vi "Transmitter HMI Main.vi"() -> ()   [LabVIEW 2025]
uses:
  Globals/Cancelled Global.vi
  Globals/Solenoid VISA Global.vi
  <vilib>/Instr/_visa.llb/VISA Configure Serial Port (Instr).vi
  Globals/Touch VISA Global.vi
  Globals/Light VISA Global.vi
  Globals/Motor VISA Global.vi
  Globals/Speaker VISA Global.vi
  Globals/Wire VISA Global.vi
  Globals/Percent Complete Global.vi
panel:
  in  "Enable Wire":bool
  in  "Enable Speaker":bool
  in  "Enable Motor":bool
  in  "Enable Light":bool
  in  "Enable Touch":bool
  in  "Enable Solenoid":bool
  in  "FREQUENCY CHANGER":bool
  in  "Speaker":bool
  in  "Wire":bool
  out "Start Transmission":bool
  out "Exit":bool
  out "Transmitting":bool
  out "Chosen Text":string
  out "Chosen Image Path":path caption="selected path"
  out "Chosen Transmission Method":u16(ring) items=["Speaker", "Wire", "Motor", "Touch", "Light", "Solenoid"]
  out "Chosen Data Type":u16(ring) items=["Text File", "Image File", "Image", "Text"]
  in  "Cancel Button":bool
  out "Transmission Progress:":dbl(slide) scale=0.0..100.0
  in  "Go":bool
  in  "Motor":bool
  in  "Touch":bool
  in  "Light":bool
  in  "Solenoid":bool
  in  "Image":bool
  in  "Text":bool
  # "TRANSMITTER"
  # "1: Select Data Type:"
  # "2: Select Method of Transmission:"
  # "3: BEGIN"
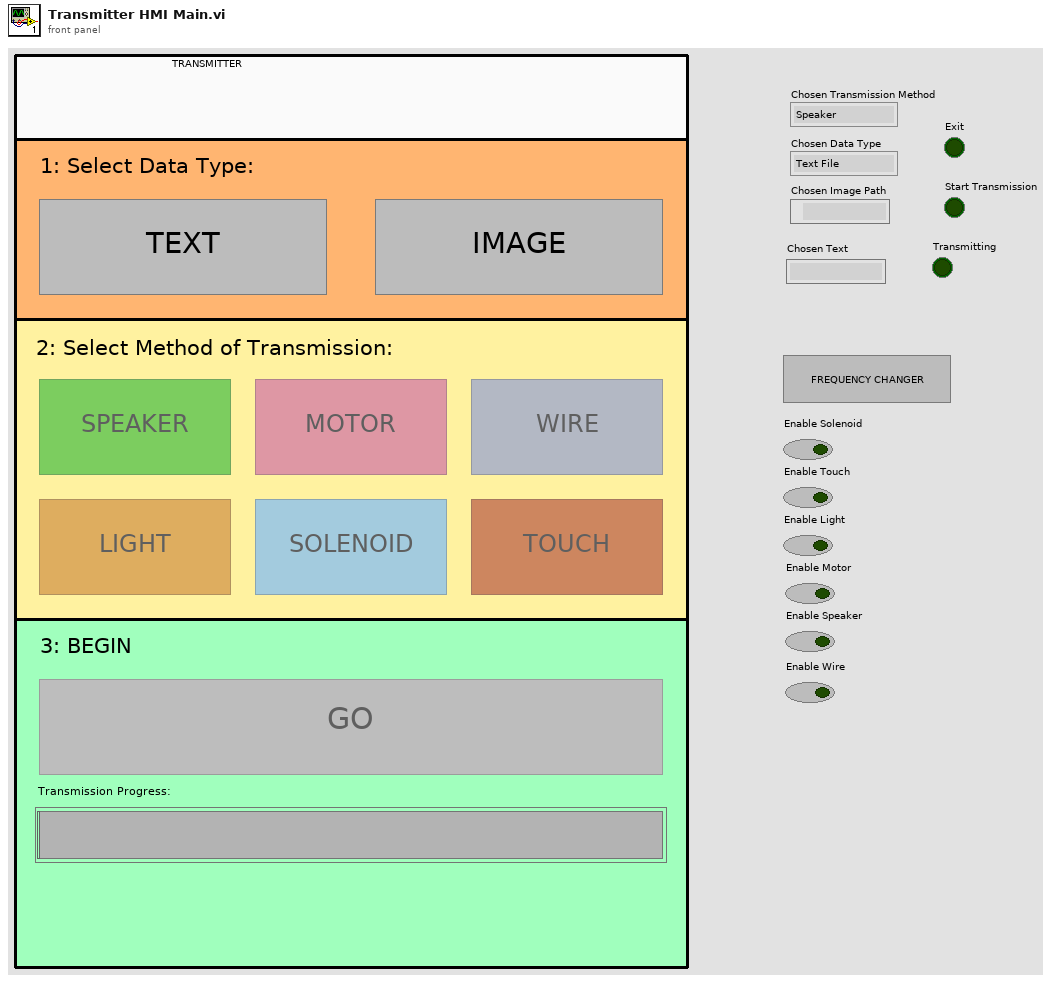
[diagram p1: front panel]
types:
  T1 = enum8{"Enabled", "Disabled", "Disabled and Grayed Out"}
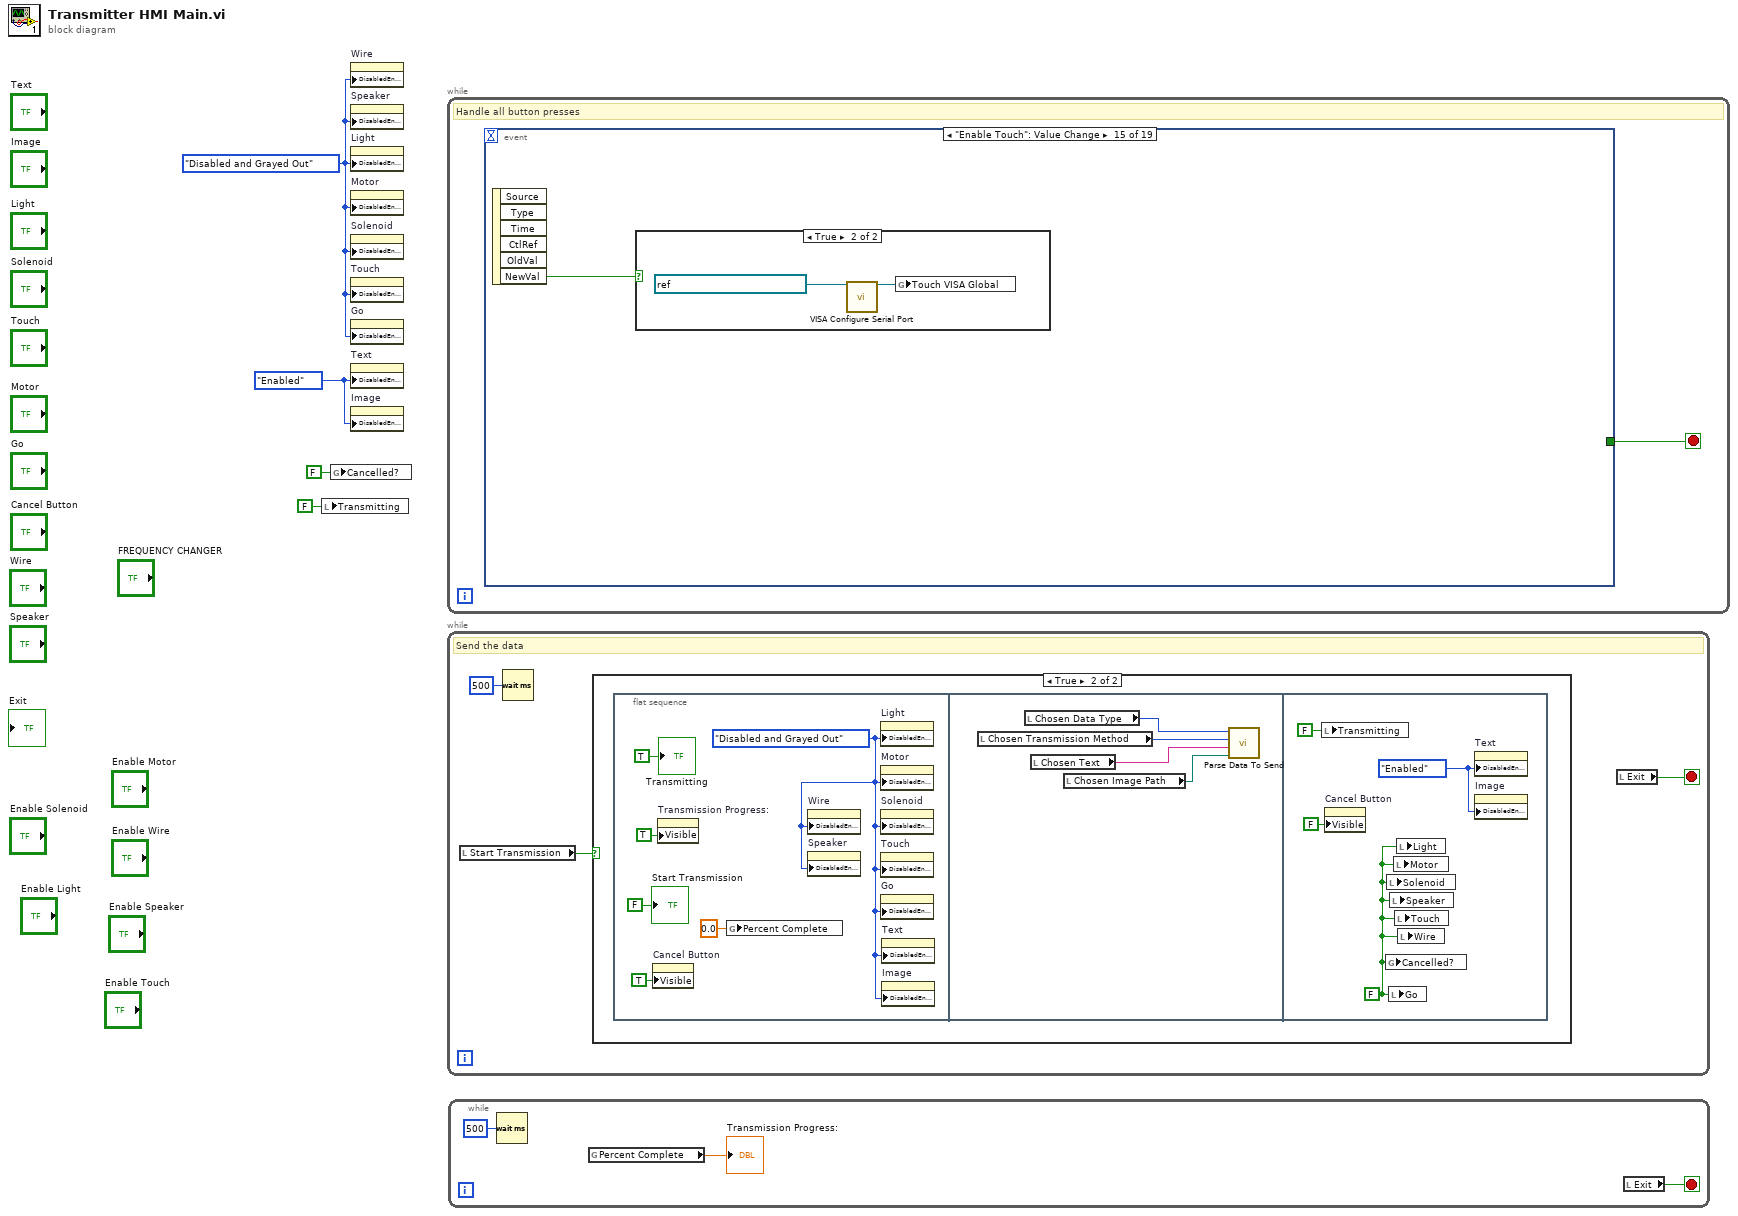
[diagram p0: block diagram]
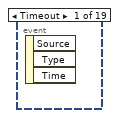
[diagram p3: hidden frame]
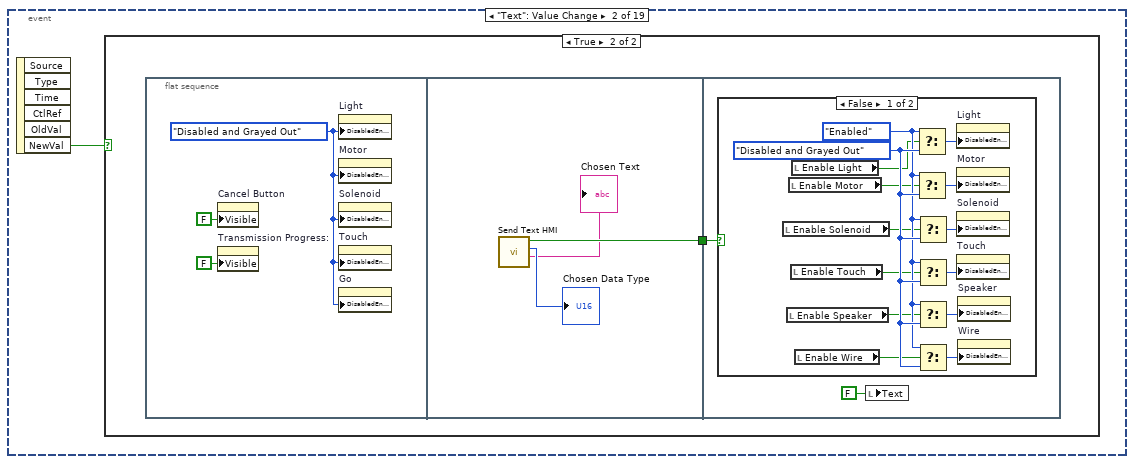
[diagram p4: hidden frame]
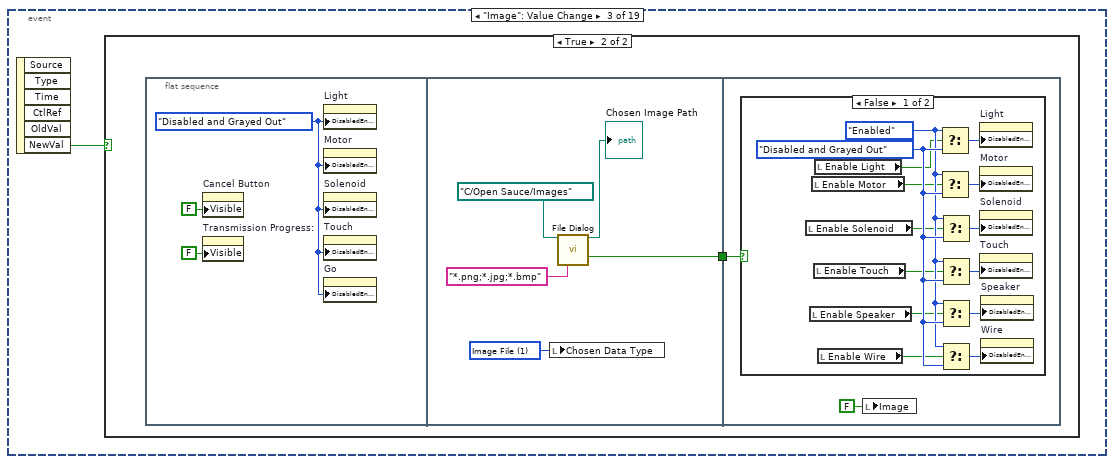
[diagram p7: hidden frame]
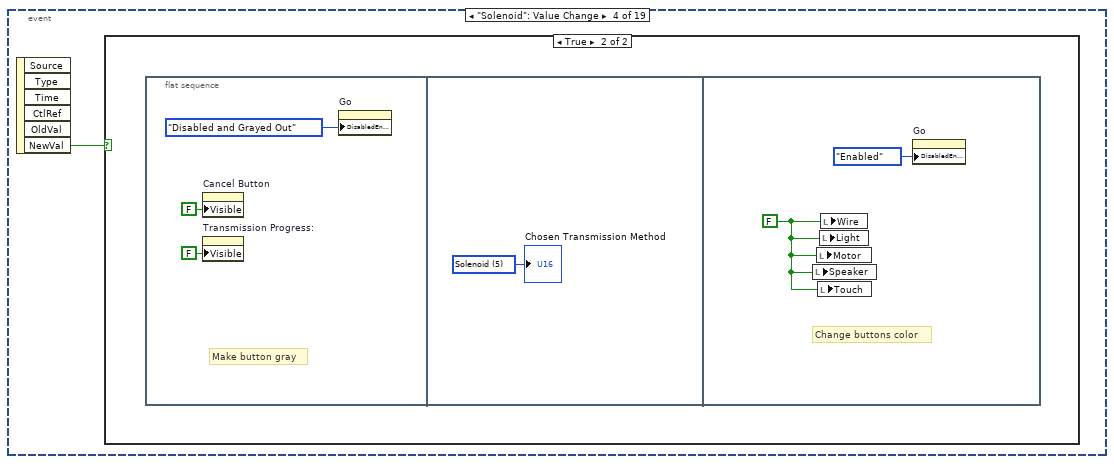
[diagram p10: hidden frame]
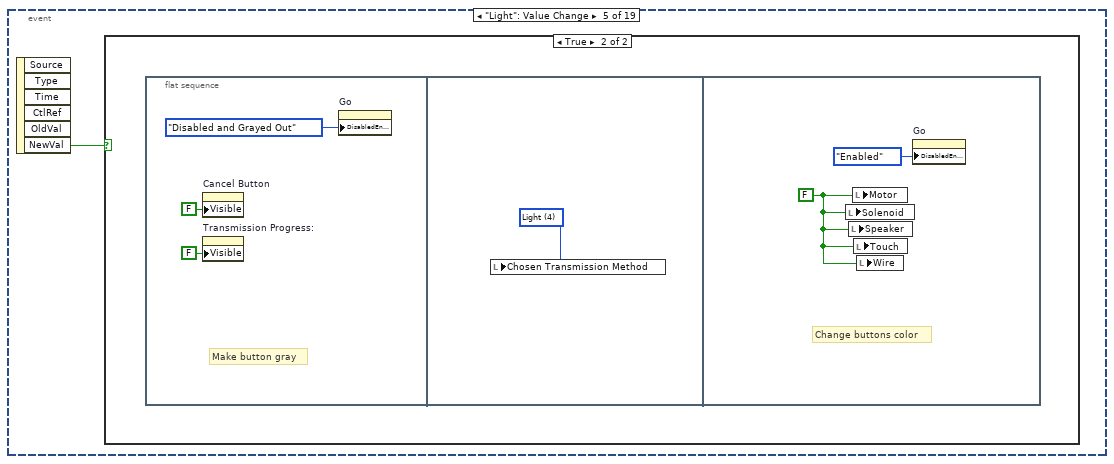
[diagram p12: hidden frame]
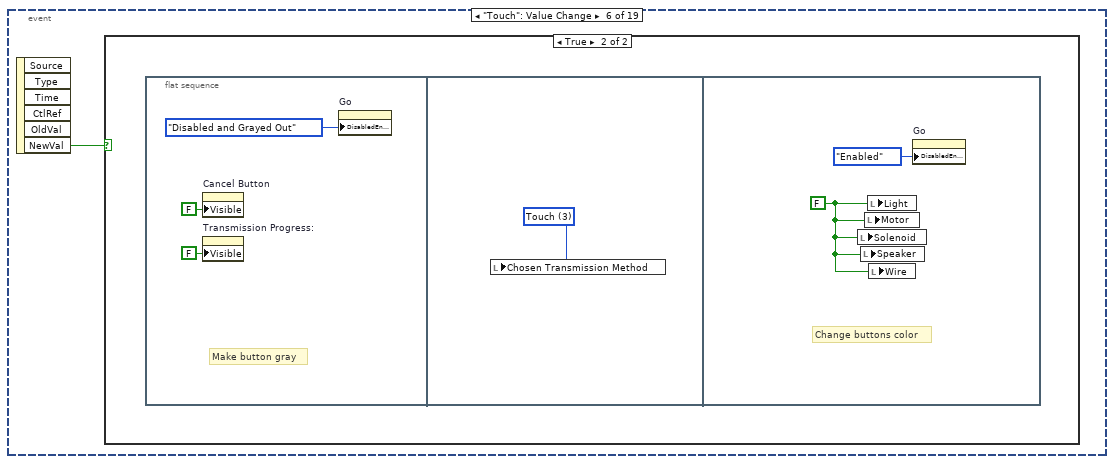
[diagram p14: hidden frame]
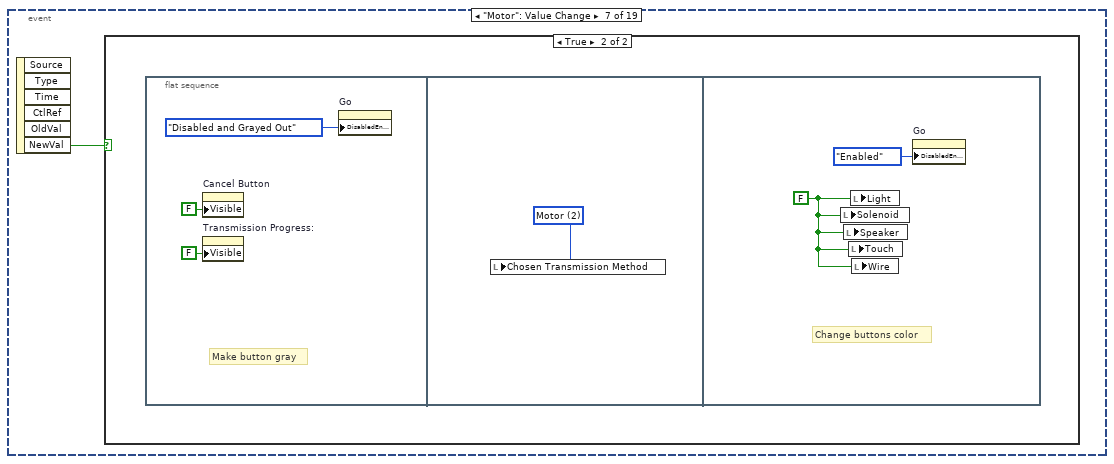
[diagram p16: hidden frame]
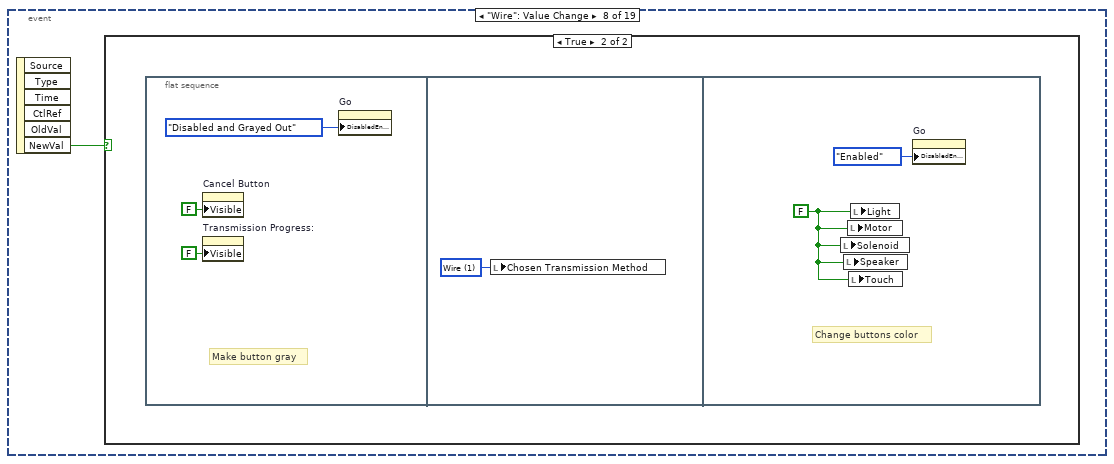
[diagram p18: hidden frame]
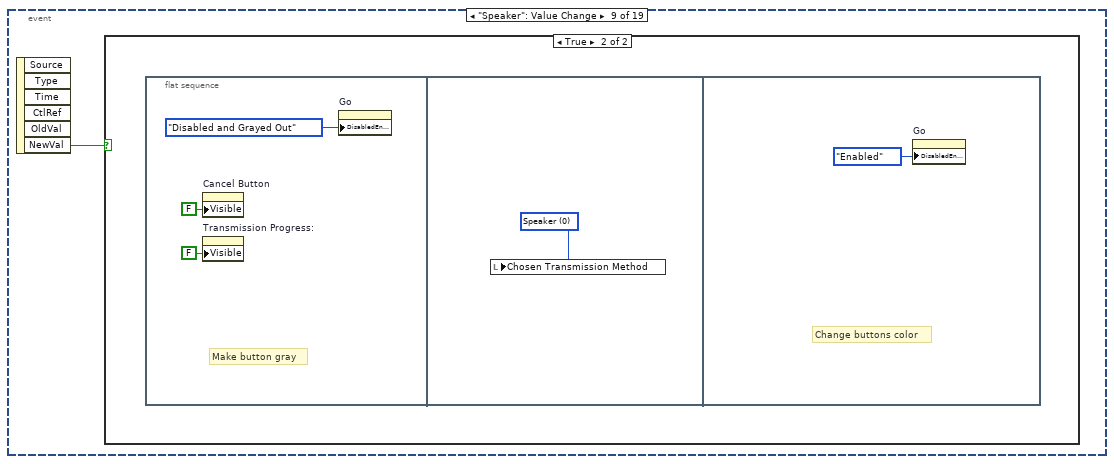
[diagram p20: hidden frame]
diagram:
  w2 = T1."Enabled" ("Disabled")
  w1 = T1."Disabled and Grayed Out" ("Disabled")
  n1 = local write "Transmitting"(FALSE ("Transmitting")) -> ()
  n2 = global write "Cancelled Global.vi" "Cancelled?"(FALSE ("Cancelled?")) -> ()
  n3 = property on="Wire" class="Bool (strict)"("DisabledEnum"=w1) -> ()  [unwired: 2 in, 2 out]
  n4 = property on="Speaker" class="Bool (strict)"("DisabledEnum"=w1) -> ()  [unwired: 2 in, 2 out]
  n5 = property on="Light" class="Bool (strict)"("DisabledEnum"=w1) -> ()  [unwired: 2 in, 2 out]
  n6 = property on="Motor" class="Bool (strict)"("DisabledEnum"=w1) -> ()  [unwired: 2 in, 2 out]
  n7 = property on="Solenoid" class="Bool (strict)"("DisabledEnum"=w1) -> ()  [unwired: 2 in, 2 out]
  n8 = property on="Touch" class="Bool (strict)"("DisabledEnum"=w1) -> ()  [unwired: 2 in, 2 out]
  n9 = property on="Go" class="Bool (strict)"("DisabledEnum"=w1) -> ()  [unwired: 2 in, 2 out]
  n10 = property on="Text" class="Bool (strict)"("DisabledEnum"=w2) -> ()  [unwired: 2 in, 2 out]
  n11 = property on="Image" class="Bool (strict)"("DisabledEnum"=w2) -> ()  [unwired: 2 in, 2 out]
  n12 = while {
    stop <- w5 stop-if-true
    # "Handle all button presses"
    n13 = event shown="[14] \"Enable Touch\": Value Change" {
      selector: _ -> [_ _ _ _ _ _ _ _ _ _ _ _ _ _ _ _ _ _ _]
      dyn-events: _ -> [_ _ _ _ _ _ _ _ _ _ _ _ _ _ _ _ _ _ _]
      timeout: _ -> [_ _ _ _ _ _ _ _ _ _ _ _ _ _ _ _ _ _ _]
      tunnel: [_ _ _ _ _ _ _ _ _ TRUE _ _ _ _ _ _ _ _ _] -> w5
      event Timeout {
        n14 = event-data() -> ()  [unwired: 1 in, 3 out]
      }
      event "Text": Value Change {
        n15 = event-data() -> ("NewVal"=w6:bool)  [unwired: 1 in, 5 out]
        n16 = case shown="True" w6 {
          frame False {
          }
          frame True {
            n17 = flat-sequence {
              tunnel: [w13] -> w7
              tunnel: w7 -> [w15]
              frame #0 {
                w9 = T1."Disabled and Grayed Out" ("Disabled")
                n18 = property on="Cancel Button" class="Bool (strict)"("Visible"=FALSE) -> ()  [unwired: 2 in, 2 out]
                n19 = property on="Transmission Progress:" class="Slide (strict)"("Visible"=FALSE) -> ()  [unwired: 2 in, 2 out]
                n20 = property on="Light" class="Bool (strict)"("DisabledEnum"=w9) -> ()  [unwired: 2 in, 2 out]
                n21 = property on="Motor" class="Bool (strict)"("DisabledEnum"=w9) -> ()  [unwired: 2 in, 2 out]
                n22 = property on="Solenoid" class="Bool (strict)"("DisabledEnum"=w9) -> ()  [unwired: 2 in, 2 out]
                n23 = property on="Touch" class="Bool (strict)"("DisabledEnum"=w9) -> ()  [unwired: 2 in, 2 out]
                n24 = property on="Go" class="Bool (strict)"("DisabledEnum"=w9) -> ()  [unwired: 2 in, 2 out]
              }
              frame #1 {
                n25 = call "Send Text HMI.vi"() -> ("Chosen Text"=→"Chosen Text":string, "Chosen Data Type"=→"Chosen Data Type":u16, "Cancelled"=w13:bool)  [unwired: 9 in]
              }
              frame #2 {
                n26 = case shown="False" w15 {
                  frame False {
                    w23 = T1."Disabled and Grayed Out" ("Disabled")
                    w22 = T1."Enabled" ("Disabled")
                    n27 = local read "Enable Solenoid"() -> (w18:bool)
                    n28 = local read "Enable Speaker"() -> (w20:bool)
                    n29 = local read "Enable Motor"() -> (w17:bool)
                    n30 = local read "Enable Touch"() -> (w19:bool)
                    n31 = local read "Enable Light"() -> (w16:bool)
                    n32 = local read "Enable Wire"() -> (w21:bool)
                    n33 = Select(t=w22, s=w16, f=w23) -> (s? t:f=w29:T1)
                    n34 = Select(t=w22, s=w17, f=w23) -> (s? t:f=w28:T1)
                    n35 = Select(t=w22, s=w18, f=w23) -> (s? t:f=w27:T1)
                    n36 = Select(t=w22, s=w19, f=w23) -> (s? t:f=w26:T1)
                    n37 = Select(t=w22, s=w20, f=w23) -> (s? t:f=w25:T1)
                    n38 = Select(t=w22, s=w21, f=w23) -> (s? t:f=w24:T1)
                    n39 = property on="Light" class="Bool (strict)"("DisabledEnum"=w29) -> ()  [unwired: 2 in, 2 out]
                    n40 = property on="Motor" class="Bool (strict)"("DisabledEnum"=w28) -> ()  [unwired: 2 in, 2 out]
                    n41 = property on="Solenoid" class="Bool (strict)"("DisabledEnum"=w27) -> ()  [unwired: 2 in, 2 out]
                    n42 = property on="Touch" class="Bool (strict)"("DisabledEnum"=w26) -> ()  [unwired: 2 in, 2 out]
                    n43 = property on="Speaker" class="Bool (strict)"("DisabledEnum"=w25) -> ()  [unwired: 2 in, 2 out]
                    n44 = property on="Wire" class="Bool (strict)"("DisabledEnum"=w24) -> ()  [unwired: 2 in, 2 out]
                  }
                  frame True {
                  }
                }
                n45 = local write "Text"(FALSE ("Text")) -> ()
              }
            }
          }
        }
      }
      event "Image": Value Change {
        n46 = event-data() -> ("NewVal"=w30:bool)  [unwired: 1 in, 5 out]
        n47 = case shown="True" w30 {
          frame False {
          }
          frame True {
            n48 = flat-sequence {
              tunnel: [w37] -> w31
              tunnel: w31 -> [w40]
              frame #0 {
                w33 = T1."Disabled and Grayed Out" ("Disabled")
                n49 = property on="Cancel Button" class="Bool (strict)"("Visible"=FALSE) -> ()  [unwired: 2 in, 2 out]
                n50 = property on="Transmission Progress:" class="Slide (strict)"("Visible"=FALSE) -> ()  [unwired: 2 in, 2 out]
                n51 = property on="Light" class="Bool (strict)"("DisabledEnum"=w33) -> ()  [unwired: 2 in, 2 out]
                n52 = property on="Motor" class="Bool (strict)"("DisabledEnum"=w33) -> ()  [unwired: 2 in, 2 out]
                n53 = property on="Solenoid" class="Bool (strict)"("DisabledEnum"=w33) -> ()  [unwired: 2 in, 2 out]
                n54 = property on="Touch" class="Bool (strict)"("DisabledEnum"=w33) -> ()  [unwired: 2 in, 2 out]
                n55 = property on="Go" class="Bool (strict)"("DisabledEnum"=w33) -> ()  [unwired: 2 in, 2 out]
              }
              frame #1 {
                w35 = u16 1 items=["Text File", "Image File", "Image", "Text"] ("Chosen Data Type")
                n56 = local write "Chosen Data Type"(w35) -> ()
                n57 = call "File Dialog"("start path"=path "C:/Open Sauce/Images", "pattern (all files)"="*.png;*.jpg;*.bmp") -> ("selected path"=→"Chosen Image Path":path, "cancelled"=w37:bool)  [unwired: 10 in, 2 out]
              }
              frame #2 {
                n58 = case shown="False" w40 {
                  frame False {
                    w49 = T1."Disabled and Grayed Out" ("Disabled")
                    w48 = T1."Enabled" ("Disabled")
                    n59 = local read "Enable Solenoid"() -> (w44:bool)
                    n60 = local read "Enable Speaker"() -> (w46:bool)
                    n61 = local read "Enable Motor"() -> (w43:bool)
                    n62 = local read "Enable Touch"() -> (w45:bool)
                    n63 = local read "Enable Light"() -> (w42:bool)
                    n64 = local read "Enable Wire"() -> (w47:bool)
                    n65 = Select(t=w48, s=w42, f=w49) -> (s? t:f=w55:T1)
                    n66 = Select(t=w48, s=w43, f=w49) -> (s? t:f=w54:T1)
                    n67 = Select(t=w48, s=w44, f=w49) -> (s? t:f=w53:T1)
                    n68 = Select(t=w48, s=w45, f=w49) -> (s? t:f=w52:T1)
                    n69 = Select(t=w48, s=w46, f=w49) -> (s? t:f=w51:T1)
                    n70 = Select(t=w48, s=w47, f=w49) -> (s? t:f=w50:T1)
                    n71 = property on="Light" class="Bool (strict)"("DisabledEnum"=w55) -> ()  [unwired: 2 in, 2 out]
                    n72 = property on="Motor" class="Bool (strict)"("DisabledEnum"=w54) -> ()  [unwired: 2 in, 2 out]
                    n73 = property on="Solenoid" class="Bool (strict)"("DisabledEnum"=w53) -> ()  [unwired: 2 in, 2 out]
                    n74 = property on="Touch" class="Bool (strict)"("DisabledEnum"=w52) -> ()  [unwired: 2 in, 2 out]
                    n75 = property on="Speaker" class="Bool (strict)"("DisabledEnum"=w51) -> ()  [unwired: 2 in, 2 out]
                    n76 = property on="Wire" class="Bool (strict)"("DisabledEnum"=w50) -> ()  [unwired: 2 in, 2 out]
                  }
                  frame True {
                  }
                }
                n77 = local write "Image"(FALSE ("Text")) -> ()
              }
            }
          }
        }
      }
      event "Solenoid": Value Change {
        n78 = event-data() -> ("NewVal"=w56:bool)  [unwired: 1 in, 5 out]
        n79 = case shown="True" w56 {
          frame False {
          }
          frame True {
            n80 = flat-sequence {
              frame #0 {
                # "Make button gray"
                n81 = property on="Cancel Button" class="Bool (strict)"("Visible"=FALSE) -> ()  [unwired: 2 in, 2 out]
                n82 = property on="Transmission Progress:" class="Slide (strict)"("Visible"=FALSE) -> ()  [unwired: 2 in, 2 out]
                n83 = property on="Go" class="Bool (strict)"("DisabledEnum"=T1."Disabled and Grayed Out" ("Disabled")) -> ()  [unwired: 2 in, 2 out]
              }
              frame #1 {
                w60 = u16 5 items=["Speaker", "Wire", "Motor", "Touch", "Light", "Solenoid"] ("Chosen Transmission Method")
                "Chosen Transmission Method" <- w60
              }
              frame #2 {
                w61 = FALSE ("Text")
                # "Change buttons color"
                n84 = local write "Speaker"(w61) -> ()
                n85 = local write "Motor"(w61) -> ()
                n86 = local write "Touch"(w61) -> ()
                n87 = local write "Light"(w61) -> ()
                n88 = local write "Wire"(w61) -> ()
                n89 = property on="Go" class="Bool (strict)"("DisabledEnum"=T1."Enabled" ("Disabled")) -> ()  [unwired: 2 in, 2 out]
              }
            }
          }
        }
      }
      event "Light": Value Change {
        n90 = event-data() -> ("NewVal"=w63:bool)  [unwired: 1 in, 5 out]
        n91 = case shown="True" w63 {
          frame False {
          }
          frame True {
            n92 = flat-sequence {
              frame #0 {
                # "Make button gray"
                n93 = property on="Cancel Button" class="Bool (strict)"("Visible"=FALSE) -> ()  [unwired: 2 in, 2 out]
                n94 = property on="Transmission Progress:" class="Slide (strict)"("Visible"=FALSE) -> ()  [unwired: 2 in, 2 out]
                n95 = property on="Go" class="Bool (strict)"("DisabledEnum"=T1."Disabled and Grayed Out" ("Disabled")) -> ()  [unwired: 2 in, 2 out]
              }
              frame #1 {
                w67 = u16 4 items=["Speaker", "Wire", "Motor", "Touch", "Light", "Solenoid"] ("Chosen Transmission Method")
                n96 = local write "Chosen Transmission Method"(w67) -> ()
              }
              frame #2 {
                w68 = FALSE ("Text")
                # "Change buttons color"
                n97 = local write "Solenoid"(w68) -> ()
                n98 = local write "Speaker"(w68) -> ()
                n99 = local write "Motor"(w68) -> ()
                n100 = local write "Touch"(w68) -> ()
                n101 = local write "Wire"(w68) -> ()
                n102 = property on="Go" class="Bool (strict)"("DisabledEnum"=T1."Enabled" ("Disabled")) -> ()  [unwired: 2 in, 2 out]
              }
            }
          }
        }
      }
      event "Touch": Value Change {
        n103 = event-data() -> ("NewVal"=w70:bool)  [unwired: 1 in, 5 out]
        n104 = case shown="True" w70 {
          frame False {
          }
          frame True {
            n105 = flat-sequence {
              frame #0 {
                # "Make button gray"
                n106 = property on="Cancel Button" class="Bool (strict)"("Visible"=FALSE) -> ()  [unwired: 2 in, 2 out]
                n107 = property on="Transmission Progress:" class="Slide (strict)"("Visible"=FALSE) -> ()  [unwired: 2 in, 2 out]
                n108 = property on="Go" class="Bool (strict)"("DisabledEnum"=T1."Disabled and Grayed Out" ("Disabled")) -> ()  [unwired: 2 in, 2 out]
              }
              frame #1 {
                w74 = u16 3 items=["Speaker", "Wire", "Motor", "Touch", "Light", "Solenoid"] ("Chosen Transmission Method")
                n109 = local write "Chosen Transmission Method"(w74) -> ()
              }
              frame #2 {
                w75 = FALSE ("Text")
                # "Change buttons color"
                n110 = local write "Solenoid"(w75) -> ()
                n111 = local write "Speaker"(w75) -> ()
                n112 = local write "Motor"(w75) -> ()
                n113 = local write "Light"(w75) -> ()
                n114 = local write "Wire"(w75) -> ()
                n115 = property on="Go" class="Bool (strict)"("DisabledEnum"=T1."Enabled" ("Disabled")) -> ()  [unwired: 2 in, 2 out]
              }
            }
          }
        }
      }
      event "Motor": Value Change {
        n116 = event-data() -> ("NewVal"=w77:bool)  [unwired: 1 in, 5 out]
        n117 = case shown="True" w77 {
          frame False {
          }
          frame True {
            n118 = flat-sequence {
              frame #0 {
                # "Make button gray"
                n119 = property on="Cancel Button" class="Bool (strict)"("Visible"=FALSE) -> ()  [unwired: 2 in, 2 out]
                n120 = property on="Transmission Progress:" class="Slide (strict)"("Visible"=FALSE) -> ()  [unwired: 2 in, 2 out]
                n121 = property on="Go" class="Bool (strict)"("DisabledEnum"=T1."Disabled and Grayed Out" ("Disabled")) -> ()  [unwired: 2 in, 2 out]
              }
              frame #1 {
                w81 = u16 2 items=["Speaker", "Wire", "Motor", "Touch", "Light", "Solenoid"] ("Chosen Transmission Method")
                n122 = local write "Chosen Transmission Method"(w81) -> ()
              }
              frame #2 {
                w82 = FALSE ("Text")
                # "Change buttons color"
                n123 = local write "Solenoid"(w82) -> ()
                n124 = local write "Speaker"(w82) -> ()
                n125 = local write "Touch"(w82) -> ()
                n126 = local write "Light"(w82) -> ()
                n127 = local write "Wire"(w82) -> ()
                n128 = property on="Go" class="Bool (strict)"("DisabledEnum"=T1."Enabled" ("Disabled")) -> ()  [unwired: 2 in, 2 out]
              }
            }
          }
        }
      }
      event "Wire": Value Change {
        n129 = event-data() -> ("NewVal"=w84:bool)  [unwired: 1 in, 5 out]
        n130 = case shown="True" w84 {
          frame False {
          }
          frame True {
            n131 = flat-sequence {
              frame #0 {
                # "Make button gray"
                n132 = property on="Cancel Button" class="Bool (strict)"("Visible"=FALSE) -> ()  [unwired: 2 in, 2 out]
                n133 = property on="Transmission Progress:" class="Slide (strict)"("Visible"=FALSE) -> ()  [unwired: 2 in, 2 out]
                n134 = property on="Go" class="Bool (strict)"("DisabledEnum"=T1."Disabled and Grayed Out" ("Disabled")) -> ()  [unwired: 2 in, 2 out]
              }
              frame #1 {
                w88 = u16 1 items=["Speaker", "Wire", "Motor", "Touch", "Light", "Solenoid"] ("Chosen Transmission Method")
                n135 = local write "Chosen Transmission Method"(w88) -> ()
              }
              frame #2 {
                w89 = FALSE ("Text")
                # "Change buttons color"
                n136 = local write "Solenoid"(w89) -> ()
                n137 = local write "Speaker"(w89) -> ()
                n138 = local write "Motor"(w89) -> ()
                n139 = local write "Touch"(w89) -> ()
                n140 = local write "Light"(w89) -> ()
                n141 = property on="Go" class="Bool (strict)"("DisabledEnum"=T1."Enabled" ("Disabled")) -> ()  [unwired: 2 in, 2 out]
              }
            }
          }
        }
      }
      event "Speaker": Value Change {
        n142 = event-data() -> ("NewVal"=w91:bool)  [unwired: 1 in, 5 out]
        n143 = case shown="True" w91 {
          frame False {
          }
          frame True {
            n144 = flat-sequence {
              frame #0 {
                # "Make button gray"
                n145 = property on="Cancel Button" class="Bool (strict)"("Visible"=FALSE) -> ()  [unwired: 2 in, 2 out]
                n146 = property on="Transmission Progress:" class="Slide (strict)"("Visible"=FALSE) -> ()  [unwired: 2 in, 2 out]
                n147 = property on="Go" class="Bool (strict)"("DisabledEnum"=T1."Disabled and Grayed Out" ("Disabled")) -> ()  [unwired: 2 in, 2 out]
              }
              frame #1 {
                w95 = u16 0 items=["Speaker", "Wire", "Motor", "Touch", "Light", "Solenoid"] ("Chosen Transmission Method")
                n148 = local write "Chosen Transmission Method"(w95) -> ()
              }
              frame #2 {
                # "Change buttons color"
                n149 = property on="Go" class="Bool (strict)"("DisabledEnum"=T1."Enabled" ("Disabled")) -> ()  [unwired: 2 in, 2 out]
              }
            }
          }
        }
      }
      event Panel Close {
        n150 = event-data() -> ()  [unwired: 1 in, 4 out]
      }
      event "Go": Value Change {
        n151 = event-data() -> ("NewVal"=w98:bool)  [unwired: 1 in, 5 out]
        n152 = case shown="True" w98 {
          frame False {
          }
          frame True {
            n153 = local write "Cancel Button"(FALSE ("Cancel Button")) -> ()
            n154 = local write "Start Transmission"(TRUE ("Start Transmission")) -> ()
          }
        }
      }
      event "Cancel Button": Value Change {
        n155 = event-data() -> ("NewVal"=w101:bool)  [unwired: 1 in, 5 out]
        n156 = global write "Cancelled Global.vi" "Cancelled?"(w101) -> ()
      }
      event "FREQUENCY CHANGER": Value Change {
        n157 = event-data() -> ("NewVal"=w102:bool)  [unwired: 1 in, 5 out]
        n158 = case shown="True" w102 {
          frame False {
          }
          frame True {
            n159 = call "Frequency Changer.vi"() -> ()  [unwired: 12 in]
            n160 = local write "FREQUENCY CHANGER"(FALSE ("FREQUENCY CHANGER")) -> ()
          }
        }
      }
      event "Enable Solenoid": Value Change {
        n161 = event-data() -> ("NewVal"=w104:bool)  [unwired: 1 in, 5 out]
        n162 = case shown="False" w104 {
          frame False {
            n163 = global read "Solenoid VISA Global.vi" "Solenoid VISA Global"() -> (w105:refnum<visa-resource-name>)
            n164 = VISA Close(VISA resource name=w105) -> ()  [unwired: 1 in, 1 out]
          }
          frame True {
            n165 = call-poly "VISA Configure Serial Port"("VISA resource name"=refnum<visa-resource-name> "SOLENOID_TRANSMITTER") -> ("VISA resource name out"=w106:refnum<visa-resource-name>)  [unwired: 13 in, 1 out]
            n166 = global write "Solenoid VISA Global.vi" "Solenoid VISA Global"(w106) -> ()
          }
        }
      }
      event "Enable Touch": Value Change {
        n167 = event-data() -> ("NewVal"=w108:bool)  [unwired: 1 in, 5 out]
        n168 = case shown="True" w108 {
          frame False {
            n169 = global read "Touch VISA Global.vi" "Touch VISA Global"() -> (w109:refnum<visa-resource-name>)
            n170 = VISA Close(VISA resource name=w109) -> ()  [unwired: 1 in, 1 out]
          }
          frame True {
            n171 = call-poly "VISA Configure Serial Port"("VISA resource name"=refnum<visa-resource-name> "TOUCH_TRANSMITTER") -> ("VISA resource name out"=w110:refnum<visa-resource-name>)  [unwired: 13 in, 1 out]
            n172 = global write "Touch VISA Global.vi" "Touch VISA Global"(w110) -> ()
          }
        }
      }
      event "Enable Light": Value Change {
        n173 = event-data() -> ("NewVal"=w112:bool)  [unwired: 1 in, 5 out]
        n174 = case shown="True" w112 {
          frame False {
            n175 = global read "Touch VISA Global.vi" "Touch VISA Global"() -> (w113:refnum<visa-resource-name>)
            n176 = VISA Close(VISA resource name=w113) -> ()  [unwired: 1 in, 1 out]
          }
          frame True {
            n177 = call-poly "VISA Configure Serial Port"("VISA resource name"=refnum<visa-resource-name> "LIGHT_TRANSMITTER") -> ("VISA resource name out"=w115:refnum<visa-resource-name>)  [unwired: 13 in, 1 out]
            n178 = global write "Light VISA Global.vi" "LIGHT VISA resource name out"(w115) -> ()
          }
        }
      }
      event "Enable Motor": Value Change {
        n179 = event-data() -> ("NewVal"=w116:bool)  [unwired: 1 in, 5 out]
        n180 = case shown="False" w116 {
          frame False {
            n181 = global read "Motor VISA Global.vi" "Motor VISA Global"() -> (w117:refnum<visa-resource-name>)
            n182 = VISA Close(VISA resource name=w117) -> ()  [unwired: 1 in, 1 out]
          }
          frame True {
            n183 = call-poly "VISA Configure Serial Port"("VISA resource name"=refnum<visa-resource-name> "MOTOR_TRANSMITTER") -> ("VISA resource name out"=w118:refnum<visa-resource-name>)  [unwired: 13 in, 1 out]
            n184 = global write "Motor VISA Global.vi" "Motor VISA Global"(w118) -> ()
          }
        }
      }
      event "Enable Speaker": Value Change {
        n185 = event-data() -> ("NewVal"=w120:bool)  [unwired: 1 in, 5 out]
        n186 = case shown="False" w120 {
          frame False {
            n187 = global read "Speaker VISA Global.vi" "Speaker VISA Global"() -> (w121:refnum<visa-resource-name>)
            n188 = VISA Close(VISA resource name=w121) -> ()  [unwired: 1 in, 1 out]
          }
          frame True {
            n189 = call-poly "VISA Configure Serial Port"("VISA resource name"=refnum<visa-resource-name> "SPEAKER_TRANSMITTER") -> ("VISA resource name out"=w122:refnum<visa-resource-name>)  [unwired: 13 in, 1 out]
            n190 = global write "Speaker VISA Global.vi" "Speaker VISA Global"(w122) -> ()
          }
        }
      }
      event "Enable Wire": Value Change {
        n191 = event-data() -> ("NewVal"=w124:bool)  [unwired: 1 in, 5 out]
        n192 = case shown="True" w124 {
          frame False {
            n193 = global read "Wire VISA Global.vi" "Wire VISA Global"() -> (w125:refnum<visa-resource-name>)
            n194 = VISA Close(VISA resource name=w125) -> ()  [unwired: 1 in, 1 out]
          }
          frame True {
            n195 = call-poly "VISA Configure Serial Port"("VISA resource name"=refnum<visa-resource-name> "WIRE_TRANSMITTER", "baud rate (9600)"=u32 57600) -> ("VISA resource name out"=w127:refnum<visa-resource-name>)  [unwired: 12 in, 1 out]
            n196 = global write "Wire VISA Global.vi" "Wire VISA Global"(w127) -> ()
          }
        }
      }
    }
  }
  n197 = while {
    stop <- w131 stop-if-true
    # "Send the data"
    n198 = local read "Start Transmission"() -> (w130:bool)
    n199 = Wait (ms)(milliseconds to wait=u32 500) -> ()  [unwired: 1 out]
    n200 = case shown="True" w130 {
      frame False {
      }
      frame True {
        n201 = flat-sequence {
          frame #0 {
            w132 = T1."Disabled and Grayed Out" ("Disabled")
            n202 = property on="Cancel Button" class="Bool (strict)"("Visible"=TRUE) -> ()  [unwired: 2 in, 2 out]
            n203 = property on="Transmission Progress:" class="Slide (strict)"("Visible"=TRUE) -> ()  [unwired: 2 in, 2 out]
            n204 = global write "Percent Complete Global.vi" "Percent Complete"(0.0 ("Percent Complete")) -> ()
            n205 = property on="Wire" class="Bool (strict)"("DisabledEnum"=w132) -> ()  [unwired: 2 in, 2 out]
            n206 = property on="Speaker" class="Bool (strict)"("DisabledEnum"=w132) -> ()  [unwired: 2 in, 2 out]
            n207 = property on="Light" class="Bool (strict)"("DisabledEnum"=w132) -> ()  [unwired: 2 in, 2 out]
            n208 = property on="Motor" class="Bool (strict)"("DisabledEnum"=w132) -> ()  [unwired: 2 in, 2 out]
            n209 = property on="Solenoid" class="Bool (strict)"("DisabledEnum"=w132) -> ()  [unwired: 2 in, 2 out]
            n210 = property on="Touch" class="Bool (strict)"("DisabledEnum"=w132) -> ()  [unwired: 2 in, 2 out]
            n211 = property on="Go" class="Bool (strict)"("DisabledEnum"=w132) -> ()  [unwired: 2 in, 2 out]
            n212 = property on="Text" class="Bool (strict)"("DisabledEnum"=w132) -> ()  [unwired: 2 in, 2 out]
            n213 = property on="Image" class="Bool (strict)"("DisabledEnum"=w132) -> ()  [unwired: 2 in, 2 out]
            "Start Transmission" <- FALSE ("Start Transmission")
            "Transmitting" <- TRUE ("Transmitting")
          }
          frame #1 {
            n214 = local read "Chosen Transmission Method"() -> (w139:u16)
            n215 = local read "Chosen Data Type"() -> (w138:u16)
            n216 = local read "Chosen Text"() -> (w140:string)
            n217 = local read "Chosen Image Path"() -> (w141:path)
            n218 = call "Parse Data To Send.vi"("Chosen Image Path"=w141, "Chosen Text"=w140, "Chosen Transmission Method"=w139, "Chosen Data Type"=w138) -> ()  [unwired: 8 in]
          }
          frame #2 {
            w142 = FALSE ("Go")
            w143 = T1."Enabled" ("Disabled")
            n219 = local write "Transmitting"(FALSE ("Transmitting")) -> ()
            n220 = property on="Cancel Button" class="Bool (strict)"("Visible"=FALSE) -> ()  [unwired: 2 in, 2 out]
            n221 = global write "Cancelled Global.vi" "Cancelled?"(w142) -> ()
            n222 = local write "Solenoid"(w142) -> ()
            n223 = local write "Go"(w142) -> ()
            n224 = local write "Speaker"(w142) -> ()
            n225 = local write "Motor"(w142) -> ()
            n226 = local write "Touch"(w142) -> ()
            n227 = local write "Light"(w142) -> ()
            n228 = local write "Wire"(w142) -> ()
            n229 = property on="Text" class="Bool (strict)"("DisabledEnum"=w143) -> ()  [unwired: 2 in, 2 out]
            n230 = property on="Image" class="Bool (strict)"("DisabledEnum"=w143) -> ()  [unwired: 2 in, 2 out]
          }
        }
      }
    }
    n231 = local read "Exit"() -> (w131:bool)
  }
  n232 = while {
    stop <- w148 stop-if-true
    n233 = Wait (ms)(milliseconds to wait=u32 500) -> ()  [unwired: 1 out]
    n234 = global read "Percent Complete Global.vi" "Percent Complete"() -> (→"Transmission Progress:":dbl)
    n235 = local read "Exit"() -> (w148:bool)
  }
